vi "LTS60_TCP_Set_Current.vi"(8 "error in (no error)":errorcluster, 10 "Beam":bool, 11 "connection ID":refnum<k5>) -> (0 "error out":errorcluster, 1 "Acknowladged":bool, 2 "Beam out":bool, 3 "connection ID out":refnum<k5>)   [LabVIEW 2019]
panel:
  out "data out":string
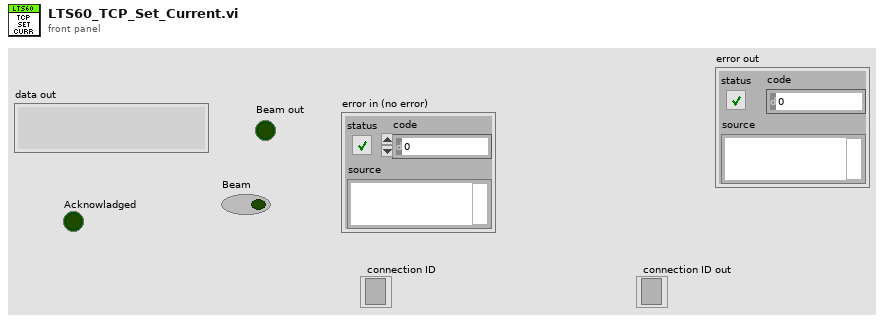
[diagram p1: front panel]
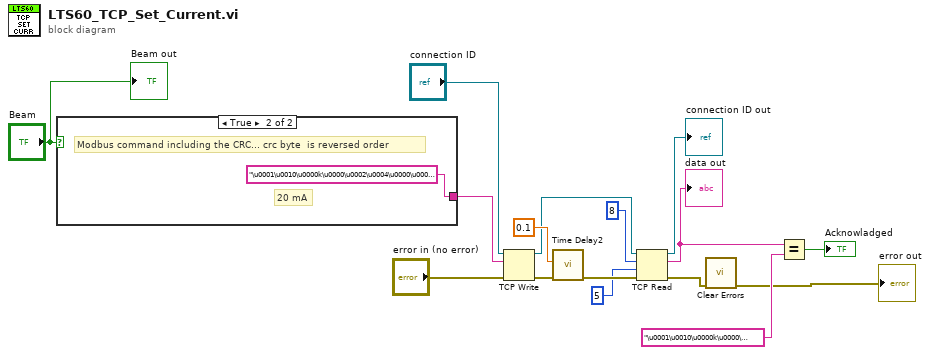
[diagram p0: block diagram]
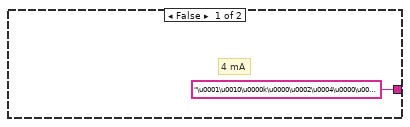
[diagram p2: hidden frame]
diagram:
  n1 = case shown="True" "Beam" {
    tunnel: ["\u0001\u0010\u0000k\u0000\u0002\u0004\u0000\u0000\u0000\u0000´4" ("write buffer") "\u0001\u0010\u0000k\u0000\u0002\u0004\u0000\u0000\u0004胺@" ("write buffer")] -> w16
    frame False {
      # "4 mA"
    }
    frame True {
      # "Modbus command including the CRC... crc byte  is reversed order"
      # "20 mA"
    }
  }
  n2 = TCP Write(connection ID="connection ID", data in=w16, error in (no error)="error in (no error)") -> (connection ID out=w12:refnum<k5>, error out=w15:errorcluster)  [unwired: 1 in, 1 out]
  n3 = call "Time Delay2"("error in (no error)"=w15, "Delay Time (s)"=0.1) -> ("error out"=w13:errorcluster)  [unwired: 9 in]
  n4 = TCP Read(connection ID=w12, bytes to read=8, error in (no error)=w13, 9:5 ("timeout ms (25000)")) -> (connection ID out=→"connection ID out":refnum<k5>, data out=w5:string, error out=w2:errorcluster)  [unwired: 1 in]
  "data out" <- w5
  n5 = call <vilib>:"Clear Errors.vi"("error in (no error)"=w2) -> ("error out"=→"error out":errorcluster)  [unwired: 5 in, 1 out]
  n6 = Equal?(x=w5, y="\u0001\u0010\u0000k\u0000\u00020\u0014" ("write buffer")) -> (x = y?=→"Acknowladged":bool)
  "Beam out" <- "Beam"
